vi "20170502127惠雨4.vi"() -> ()   [LabVIEW 2017]
uses:
  <vilib>/Utility/file.llb/Write Delimited Spreadsheet (string).vi
  <vilib>/Utility/file.llb/Write Delimited Spreadsheet (DBL).vi
panel:
  out "波形图":dbl[][](graph)
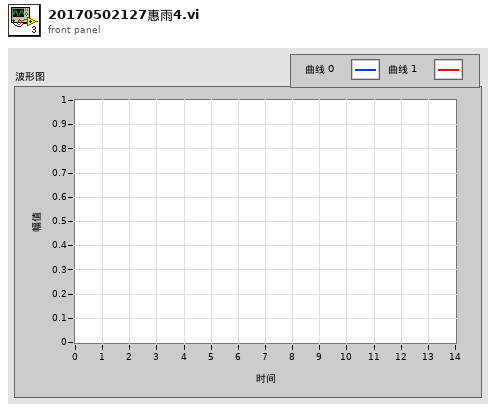
[diagram p1: front panel]
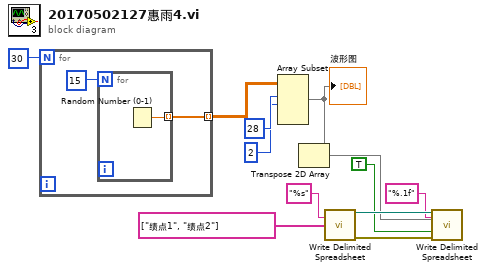
[diagram p0: block diagram]
diagram:
  n1 = for {
    N: 30 -> [_]
    tunnel: [w13] -> w11 mode=indexing
    n2 = for {
      N: 15 -> [_]
      tunnel: [w15] -> w13 mode=indexing
      n3 = Random Number (0-1)() -> (number: 0 to 1=w15:dbl)
    }
  }
  n4 = Array Subset(array=w11, index (row)=28 ("索引"), length (row)=2 ("长度")) -> (w2:dbl[][])  [unwired: 2 in]
  "波形图" <- w2
  n5 = Transpose 2D Array(2D array=w2) -> (transposed array=w1:dbl[][])
  n6 = call-poly <vilib>:"Write Delimited Spreadsheet.vi"("format (%s)"="%s" ("format (%.3f)"), "1D data"=string[] ["绩点1", "绩点2"]) -> ("new file path (Not A Path if cancelled)"=w6:path, "error out"=w5:errorcluster)  [unwired: 12 in]
  n7 = call-poly <vilib>:"Write Delimited Spreadsheet.vi"("file path (dialog if empty)"=w6, "format (%.3f)"="%.1f", "2D data"=w1, "append to file? (new file:F)"=TRUE, "error in (no error)"=w5) -> ()  [unwired: 9 in, 2 out]
